vi "_Publish Group.vi"(8 "error in (no error)":errorcluster, 10 "Group Name":string, 11 "Loop Data In":T1 {"Published Groups"."Publish Address" format="%.0x"; "Published Groups"."Last Publish" format="%<%H:%M:%S%3u>T"}) -> (0 "error out":errorcluster, 3 "Loop Data":T1 {"Published Groups"."Publish Address" format="%.0x"; "Published Groups"."Last Publish" format="%<%H:%M:%S%3u>T"})   [LabVIEW 2020, in "Vecto.lvlib" / "RemoteDataService.lvclass"]
uses:
  RemoteDataService.lvclass
  Loop Data.ctl
  SequenceCountService/SequenceCountService.lvclass
  Published Group.ctl
  Group/Group.lvclass
  Timestamp ms.vi
  proto/GroupData/Class/Msg.lvclass
  C:/Program Files (x86)/National Instruments/LabVIEW 2024/vi.lib/IlluminatedG/IG Protoc/LV-Proto/Message/Message.lvclass
  SequenceCountService/Next.vi
  proto/UdpPayload/Flatten.vi
  <vilib>/IlluminatedG/IG Protoc/LV-Proto/Message/Message.lvclass
  Vecto.lvlib
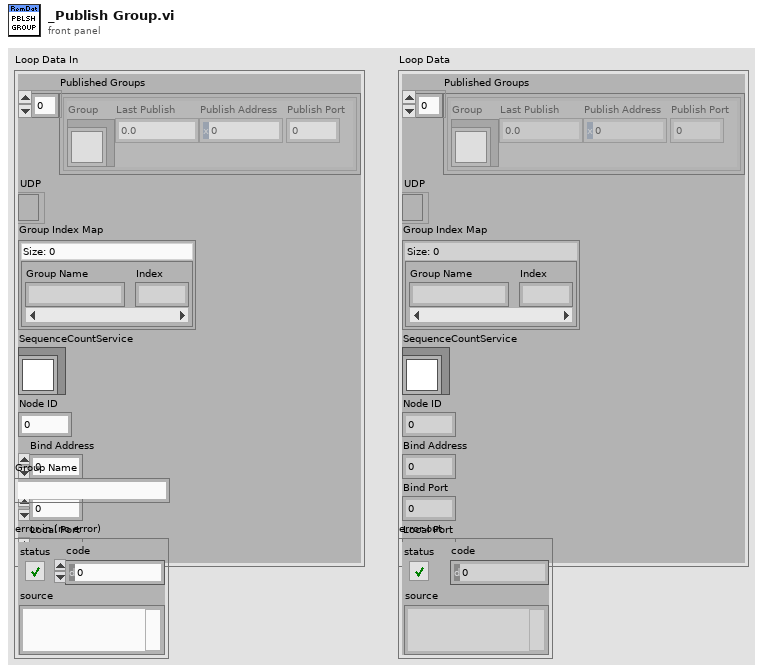
[diagram p1: front panel]
types:
  T1 = typedef "Vecto.lvlib/RemoteDataService.lvclass/Loop Data.ctl" = cluster{"Published Groups":T2[], "UDP":refnum<k16>, "Group Index Map":map{string, i32}, "SequenceCountService":refnum<class "SequenceCountService.lvclass">, "Node ID":u32, "Bind Address":u32, "Bind Port":u16, "Local Port":u16}
  T2 = typedef "Vecto.lvlib/RemoteDataService.lvclass/Published Group.ctl" = cluster{"Group":refnum<class "Group.lvclass">, "Last Publish":dbl, "Publish Address":u32, "Publish Port":u16}
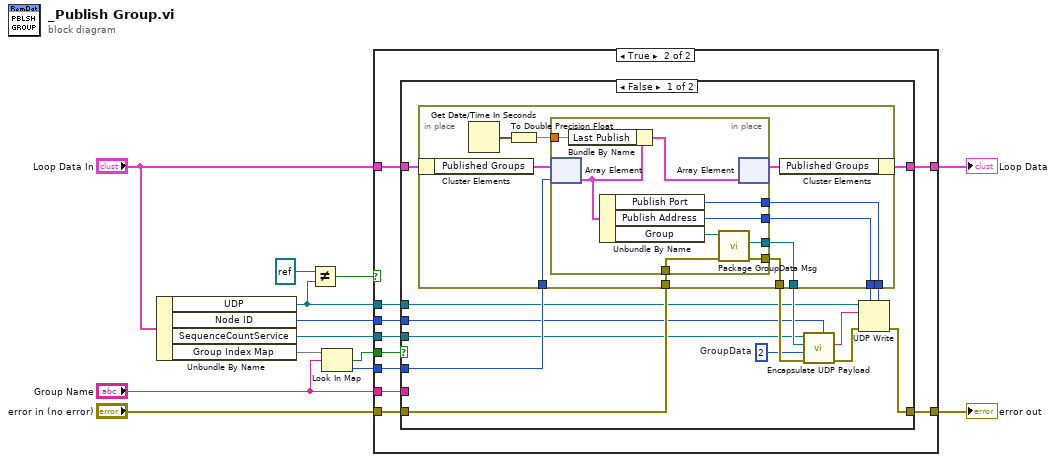
[diagram p0: block diagram]
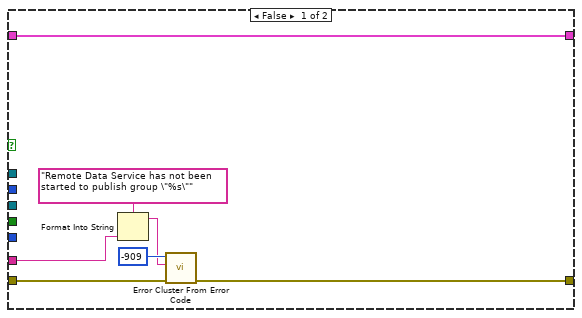
[diagram p2: hidden frame]
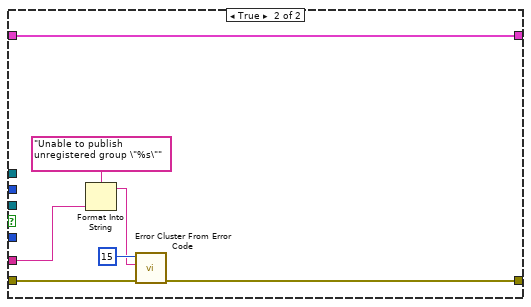
[diagram p3: hidden frame]
diagram:
  n1 = Unbundle By Name("Loop Data In") -> ("UDP"=w3:refnum<k16>, "Node ID"=w4:u32, "SequenceCountService"=w10:refnum<class "SequenceCountService.lvclass">, "Group Index Map"=w13:map{string, i32})
  n2 = Not Equal?(x=refnum<k16> refnum, y=w3) -> (x != y?=w1:bool)
  n3 = Look In Map(map=w13, key="Group Name") -> (key not found?=w12:bool, value=w11:i32)  [unwired: 1 in]
  n4 = case shown="True" w1 {
    tunnel: w12 -> [_ w30]
    tunnel: w11 -> [_ w29]
    tunnel: w10 -> [_ w28]
    tunnel: "Loop Data In" -> [w20 w27]
    tunnel: "error in (no error)" -> [w19 w26]
    tunnel: "Group Name" -> [w15 w25]
    tunnel: [w20 w24] -> w6
    tunnel: [w18 w23] -> w5
    tunnel: w4 -> [_ w22]
    tunnel: w3 -> [_ w21]
    frame False {
      n5 = Format Into String(format string="Remote Data Service has not been started to publish group \"%s\"", w15) -> (resulting string=w14:string)  [unwired: 2 in, 1 out]
      n6 = call <vilib>:"Error Cluster From Error Code.vi"("error in (no error)"=w19, "error message (\"\")"=w14, "error code (0)"=-909) -> ("error out"=w18:errorcluster)  [unwired: 6 in]
    }
    frame True {
      n7 = case shown="False" w30 {
        tunnel: w29 -> [w41 _]
        tunnel: w28 -> [w39 _]
        tunnel: w27 -> [w43 w66]
        tunnel: w26 -> [w45 w71]
        tunnel: w25 -> [_ w69]
        tunnel: [w42 w66] -> w24
        tunnel: [w34 w65] -> w23
        tunnel: w22 -> [w37 _]
        tunnel: w21 -> [w36 _]
        frame False {
          w38 = u32 2  # GroupData
          n8 = in-place {
            in-place-border: w41 -> [w53]
            in-place-border: [w50] -> w40
            in-place-border: [w49] -> w44
            in-place-border: [w48] -> w32
            in-place-border: [w47] -> w31
            in-place-border: w45 -> [w46]
            n9 = in-place-cluster #1(w43) -> ("Published Groups"=w55:T2[])
            n10 = Get Date/Time In Seconds() -> (seconds since 1Jan1904=w52:timestamp)
            n11 = To Double Precision Float(number=w52) -> (double precision float=w51:dbl)
            n12 = in-place {
              in-place-border: w51 -> [w63]
              in-place-border: [w60] -> w50
              in-place-border: [w59] -> w49
              in-place-border: [w58] -> w48
              in-place-border: [w57] -> w47
              in-place-border: w46 -> [w56]
              n13 = in-place-array #2(w55, w53) -> (w62:T2)
              n14 = Bundle By Name(cluster=w62, "Last Publish"=w63) -> (w64:T2)
              n15 = Unbundle By Name(w62) -> ("Publish Port"=w57:u16, "Publish Address"=w58:u32, "Group"=w61:refnum<class "Group.lvclass">)
              n16 = call "Package GroupData Msg.vi"("error in (no error)"=w56, "Group in"=w61) -> ("error out"=w59:errorcluster, "GroupData Msg"=w60:refnum<class "Msg.lvclass">)  [unwired: 7 in, 1 out]
              n17 = in-place-array #2(w64) -> (w54:T2[])  [unwired: 1 out]
            }
            n18 = in-place-cluster #1("Published Groups"=w54) -> (w42:T1)
          }
          n19 = call "Encapsulate UDP Payload.vi"("source_id"=w37, "error in (no error)"=w44, "type_id"=w38, "Encapsulated Msg"=w40, "SequenceCountService"=w39) -> ("error out"=w35:errorcluster, "UDP Payload"=w33:string)  [unwired: 5 in]
          n20 = UDP Write(address=w32, port or service name=w31, connection ID=w36, data in=w33, 8:w35) -> (error out=w34:errorcluster)  [unwired: 1 in, 1 out]
        }
        frame True {
          n21 = Format Into String(format string="Unable to publish unregistered group \"%s\"", w69) -> (resulting string=w67:string)  [unwired: 2 in, 1 out]
          n22 = call <vilib>:"Error Cluster From Error Code.vi"("error in (no error)"=w71, "error message (\"\")"=w67, "error code (0)"=15) -> ("error out"=w65:errorcluster)  [unwired: 6 in]
        }
      }
    }
  }
  "Loop Data" <- w6
  "error out" <- w5
